vi "iterate.vi"(8 "error in (no error)":errorcluster, 11 "MG090623BinningImageAssembler in":refnum<class "ImageAssemblerMG090623Binning.lvclass">) -> (0 "error out":errorcluster, 2 "finished?":bool, 3 "MG090623BinningImageAssembler out":refnum<class "ImageAssemblerMG090623Binning.lvclass">)   [LabVIEW 2010, in "ImageAssemblerMG090623Binning.lvclass"]
uses:
  ImageAssemblerMG090623Binning.lvclass
  common/classes/Image/Image/Image.lvclass
  ImageAssemblerMG090623Binning.lvclass/ImageAssemblerMG090623Binning.ctl
  common/classes/ErrorController/ErrorController/class_data.vi
  ImageAssemblerDL090211Scaffold/ImageAssemblerDL090211Scaffold/ImageAssemblerDL090211Scaffold.lvclass
  common/classes/ErrorController/ErrorController/ErrorController.lvclass
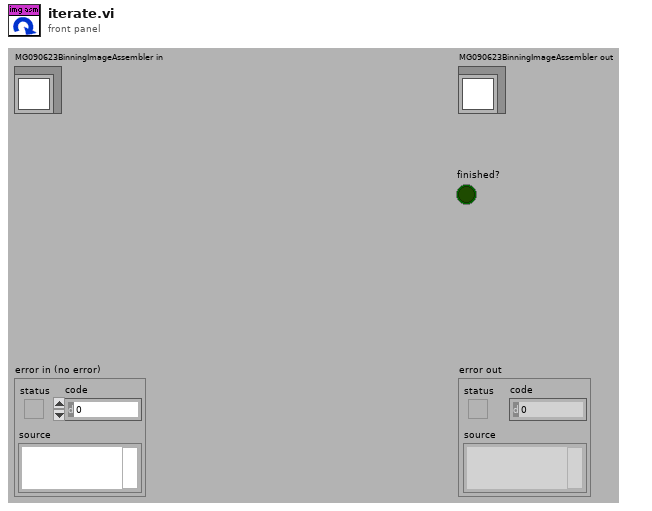
[diagram p1: front panel]
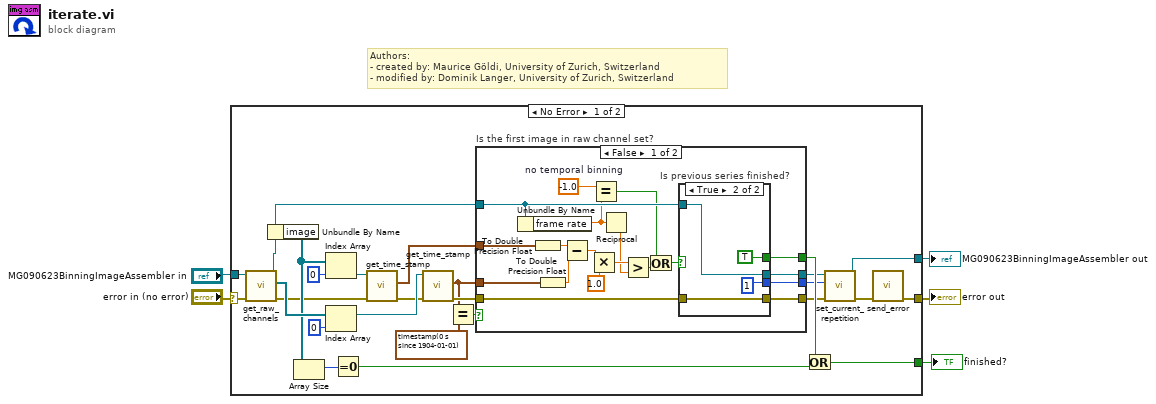
[diagram p0: block diagram]
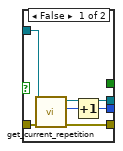
[diagram p2: hidden frame]
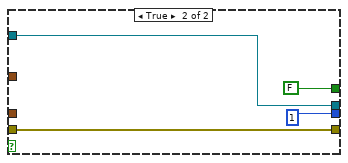
[diagram p3: hidden frame]
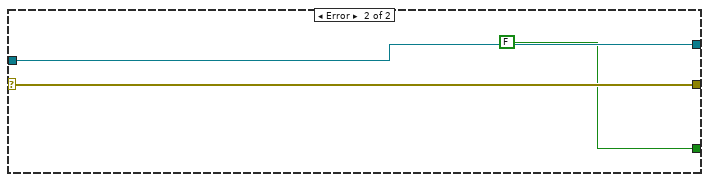
[diagram p4: hidden frame]
diagram:
  # "Authors: \n- created by: Maurice Göldi, University of Zurich, Switzerland\n- modified by: Dominik Langer, University of Zurich, Switzerland"
  n1 = case shown="No Error" "error in (no error)" {
    selector: "error in (no error)" -> [w26 w67]
    tunnel: [w6 w67] -> w1
    tunnel: [w9 w66] -> w2
    tunnel: "MG090623BinningImageAssembler in" -> [w24 w66]
    tunnel: [w16 FALSE] -> w3
    frame No Error {
      n2 = call-dynamic "get_raw_channels.vi"("error in (no error)"=w26, "DL090211ImageAssemblerScaffold.lvclass in"=w24) -> ("error out"=w12:errorcluster, "raw channels"=w22:refnum<class "Image.lvclass">[], "DL090211ImageAssemblerScaffold.lvclass out"=w13:refnum<class "ImageAssemblerMG090623Binning.lvclass">)  [unwired: 7 out]
      n3 = Unbundle By Name(w13) -> ("image"=w14:refnum<class "Image.lvclass">[])
      n4 = Array Size(array=w14) -> (size(s)=w18:i32)
      n5 = Index Array(array=w14, index=0) -> (element=w31:refnum<class "Image.lvclass">)
      n6 = Index Array(array=w22, index=0) -> (element=w28:refnum<class "Image.lvclass">)
      n7 = Equal To 0?(x=w18) -> (x = 0?=w17:bool)
      n8 = call-dynamic "get_time_stamp.vi"("error in (no error)"=w12, "Image.lvclass in"=w31) -> ("error out"=w27:errorcluster, "timestamp"=w25:timestamp)  [unwired: 8 out]
      n9 = call-dynamic "get_time_stamp.vi"("error in (no error)"=w27, "Image.lvclass in"=w28) -> ("error out"=w23:errorcluster, "timestamp"=w21:timestamp)  [unwired: 8 out]
      n10 = Equal?(x=w21, y=timestamp(0 s since 1904-01-01)) -> (x = y?=w19:bool)
      n11 = case "Is the first image in raw channel set?" shown="False" w19 {
        tunnel: [w50 FALSE] -> w15
        tunnel: w25 -> [w43 _]
        tunnel: w13 -> [w42 w62]
        tunnel: [w41 w62] -> w8
        tunnel: w23 -> [w40 w61]
        tunnel: [w39 w61] -> w10
        tunnel: w21 -> [w38 _]
        tunnel: [w37 1 ("current repetition")] -> w11
        frame False {
          w35 = dbl[unit] -1.0  # no temporal binning
          n12 = Unbundle By Name(w42) -> ("frame rate"=w36:dbl[unit])
          n13 = To Double Precision Float(number=w43) -> (double precision float=w46:dbl)
          n14 = To Double Precision Float(number=w38) -> (double precision float=w45:dbl)
          n15 = Subtract(x=w46, y=w45) -> (x-y=w48:dbl)
          n16 = Multiply(x=w48, y=dbl[unit] 1.0) -> (x*y=w49:dbl[unit])
          n17 = Equal?(x=w35, y=w36) -> (x = y?=w34:bool)
          n18 = Reciprocal(x=w36) -> (1/x=w44:dbl[unit])
          n19 = Greater?(x=w49, y=w44) -> (0:w33:bool)
          n20 = Or(x=w34, y=w33) -> (x .or. y?=w32:bool)
          n21 = case "Is previous series finished?" shown="True" w32 {
            tunnel: [_ TRUE] -> w50
            tunnel: w42 -> [w55 w57]
            tunnel: [w52 w57] -> w41
            tunnel: w40 -> [w54 w59]
            tunnel: [w51 w59] -> w39
            tunnel: [w53 1 ("current repetition")] -> w37
            frame False {
              n22 = call "get_current_repetition.vi"("error in (no error)"=w54, "DL090211ImageAssemblerScaffold.lvclass in"=w55) -> ("error out"=w51:errorcluster, "current repetition"=w56:i32, "DL090211ImageAssemblerScaffold.lvclass out"=w52:refnum<class "ImageAssemblerMG090623Binning.lvclass">)  [unwired: 7 in]
              n23 = Increment(x=w56) -> (x+1=w53:i32)
            }
            frame True {
            }
          }
        }
        frame True {
        }
      }
      n24 = Or(x=w15, y=w17) -> (x .or. y?=w16:bool)
      n25 = call-dynamic "set_current_repetition.vi"("error in (no error)"=w10, "current repetition"=w11, "DL090211ImageAssemblerScaffold.lvclass in"=w8) -> ("error out"=w7:errorcluster, "DL090211ImageAssemblerScaffold.lvclass out"=w9:refnum<class "ImageAssemblerMG090623Binning.lvclass">)  [unwired: 7 out]
      n26 = call "send_error.vi"("error in (no error)"=w7) -> ("error out"=w6:errorcluster)  [unwired: 10 in]
    }
    frame Error {
    }
  }
  "error out" <- w1
  "MG090623BinningImageAssembler out" <- w2
  "finished?" <- w3
